vi "Vision Server Restart ADB.vi"(1 "error in":errorcluster, 2 "Vision Server":T1={"connection ID"=refnum, "Running?"=TRUE, "TCP Port"=65535, "LastMessageReceivedTime"=0.0, "WantsAppRestart"=FALSE, "IsConnect"=FALSE, "Targets Updates"=[{"Valid?"=FALSE, "CapturedAtTimestamp"=0.0, "Targets Message"={"capturedAgoMs"=0, "targets"=[{"x"=0.0, "y"=0.0, "z"=0.0, "theta"=0.0}]}}]}) -> (0 "error out":errorcluster)   [LabVIEW 2016]
uses:
  Vision Server.ctl
  Messages/Targets/Targets Update.ctl
  Messages/Targets/Targets Message.ctl
  Messages/Targets/Targets Info.ctl
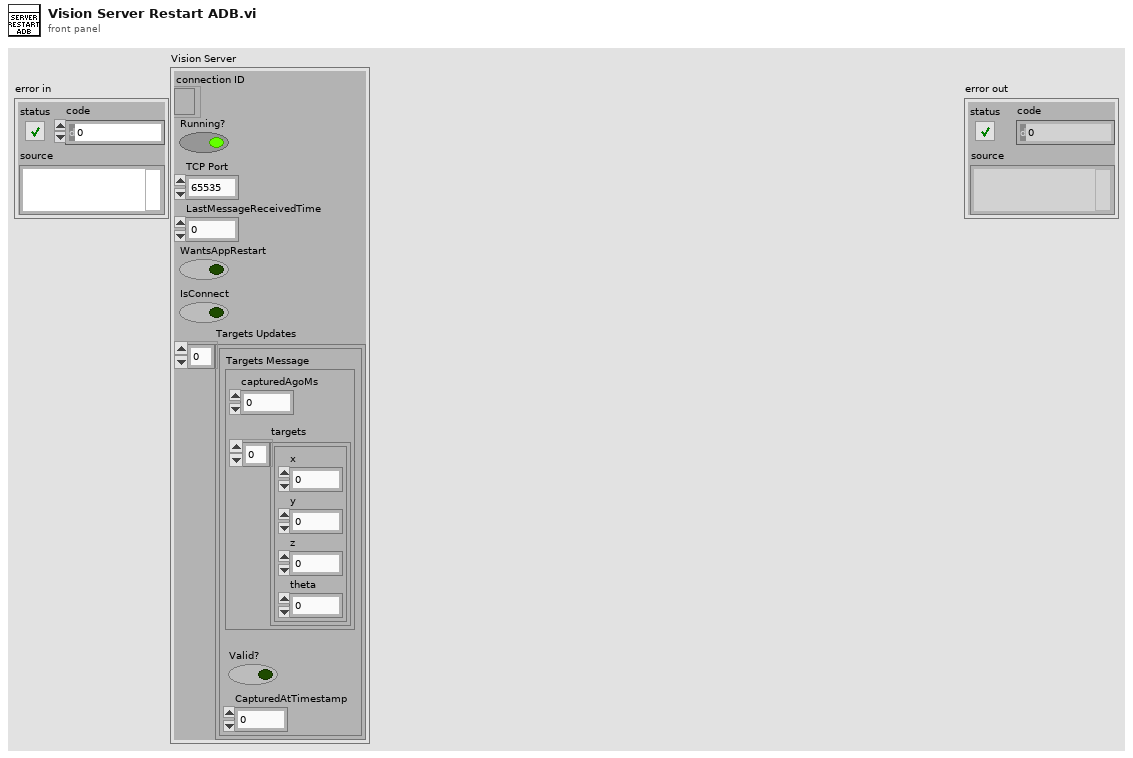
[diagram p1: front panel]
types:
  T1 = typedef "Vision Server.ctl" = cluster{"connection ID":refnum<k5>, "Running?":bool, "TCP Port":u16, "LastMessageReceivedTime":dbl, "WantsAppRestart":bool, "IsConnect":bool, "Targets Updates":T2[]}
  T2 = typedef "Targets Update.ctl" = cluster{"Valid?":bool, "CapturedAtTimestamp":dbl, "Targets Message":T3}
  T3 = typedef "Targets Message.ctl" = cluster{"capturedAgoMs":i32, "targets":T4[]}
  T4 = typedef "Targets Info.ctl" = cluster{"x":dbl, "y":dbl, "z":dbl, "theta":dbl}
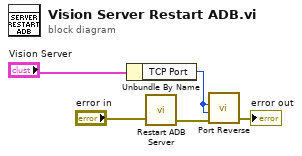
[diagram p0: block diagram]
diagram:
  n1 = Unbundle By Name("Vision Server") -> ("TCP Port"=w4:u16)
  n2 = call "Restart ADB Server.vi"("error in"="error in") -> ("error out"=w3:errorcluster)  [unwired: 3 in]
  n3 = call "Port Reverse.vi"("error in"=w3, "local TCP port"=w4, "remote TCP port"=w4) -> ("error out"=→"error out":errorcluster)  [unwired: 3 in]
